vi "Limit Switches.vi"(1 "Mode":enum8{"Start", "Run", "Finish"}(ring)) -> (0 "Limit Switches":T1)   [LabVIEW 2014]
uses:
  <vilib>/Rock Robotics/SystemInterfaces/DIO/FPGA_DIOChannel.ctl
  <vilib>/Rock Robotics/SystemInterfaces/AI/FPGA_AIChannel.ctl
panel:
  out "Voltage":dbl
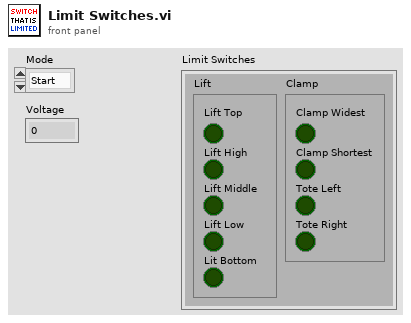
[diagram p1: front panel]
types:
  T1 = cluster{"Lift":cluster{"Lift Top":bool, "Lift High":bool, "Lift Middle":bool, "Lift Low":bool, "Lit Bottom":bool}, "Clamp":cluster{"Clamp Widest":bool, "Clamp Shortest":bool, "Tote Left":bool, "Tote Right":bool}}
  T2 = typedef "FPGA_AIChannel.ctl" = enum8{"AI 0", "AI 1", "AI 2", "AI 3", "AI MXP 0", "AI MXP 1", "AI MXP 2", "AI MXP 3", "Invalid"}
  T3 = typedef "FPGA_DIOChannel.ctl" = enum8{"DIO 0", "DIO 1", "DIO 2", "DIO 3", "DIO 4", "DIO 5", "DIO 6", "DIO 7", "DIO 8", "DIO 9", "DIO MXP 0", "DIO MXP 1", "DIO MXP 2", "DIO MXP 3", "DIO MXP 4", "DIO MXP 5", "DIO MXP 6", "DIO MXP 7", "DIO MXP 8", "DIO MXP 9", "DIO MXP 10", "DIO MXP 11", "DIO MXP 12", "DIO MXP 13", "DIO MXP 14", "DIO MXP 15", "Invalid"}
  T4 = typedef "WPI_AnalogChannelDevRef.ctl" = cluster{"DevStatus":errorcluster, "Controller":T5, "Analog Channel":T2}
  T5 = typedef "FPGA_TypedefAnalogModule.ctl" = enum16{"Controller 1"}
  T6 = typedef "WPI_DigitalInputDevRef.ctl" = cluster{"DevStatus":errorcluster, "DIO Channel":T3, "Controller":T7}
  T7 = typedef "FPGA_TypedefDigitalModule.ctl" = enum16{"Controller 1"}
  T8 = cluster{"Value":bool, "Value":bool, "Value":bool, "Value":bool}
  T9 = cluster{cluster{bool, bool, bool, bool, bool}, cluster{"Value":bool, "Value":bool, "Value":bool, "Value":bool}}
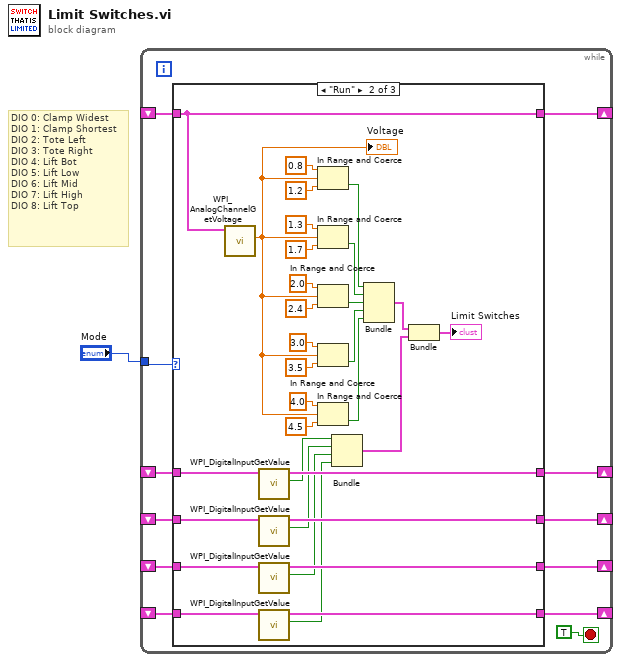
[diagram p0: block diagram]
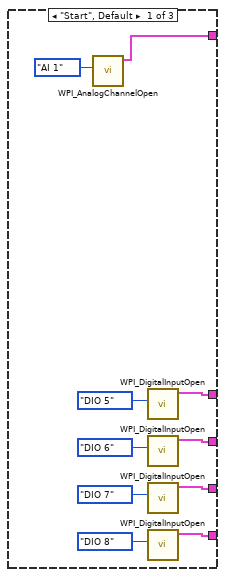
[diagram p2: hidden frame]
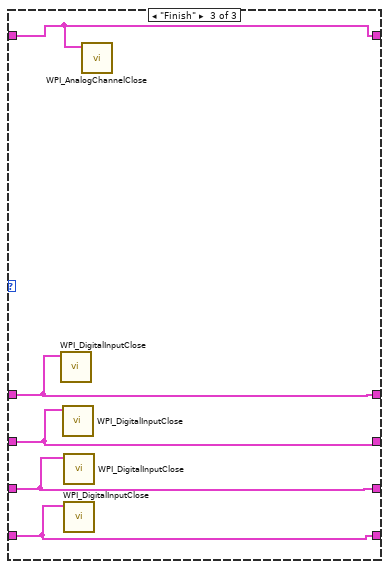
[diagram p3: hidden frame]
diagram:
  # "DIO 0: Clamp Widest\nDIO 1: Clamp Shortest\nDIO 2: Tote Left\nDIO 3: Tote Right\nDIO 4: Lift Bot\nDIO 5: Lift Low\nDIO 6: Lift Mid\nDIO 7: Lift High\nDIO 8: Lift Top"
  n1 = while {
    tunnel: "Mode" -> [w13]
    shift-right: [w12] -> _
    shift-left: _ -> [w11]
    shift-right: [w9] -> _
    shift-left: _ -> [w5]
    shift-right: [w8] -> _
    shift-left: _ -> [w4]
    shift-right: [w7] -> _
    shift-left: _ -> [w3]
    shift-right: [w6] -> _
    shift-left: _ -> [w2]
    stop <- TRUE stop-if-true
    n2 = case shown="\"Run\"" w13 {
      tunnel: [w14 w41 w56] -> w12
      tunnel: w11 -> [_ w41 w56]
      tunnel: [w19 w51 w60] -> w9
      tunnel: [w18 w50 w59] -> w8
      tunnel: [w17 w49 w58] -> w7
      tunnel: [w16 w48 w57] -> w6
      tunnel: w5 -> [_ w55 w60]
      tunnel: w4 -> [_ w54 w59]
      tunnel: w3 -> [_ w53 w58]
      tunnel: w2 -> [_ w52 w57]
      frame "Start", Default {
        n3 = call <vilib>:"WPI_AnalogChannelOpen.vi"("Analog Channel"=FPGA_AIChannel."AI 1") -> ("AIDeviceRef"=w14:T4)  [unwired: 9 in, 1 out]
        n4 = call <vilib>:"WPI_DigitalInputOpen.vi"("DIO Channel"=FPGA_DIOChannel."DIO 5") -> ("DigitalInputDevRef"=w19:T6)  [unwired: 9 in, 1 out]
        n5 = call <vilib>:"WPI_DigitalInputOpen.vi"("DIO Channel"=FPGA_DIOChannel."DIO 6") -> ("DigitalInputDevRef"=w18:T6)  [unwired: 9 in, 1 out]
        n6 = call <vilib>:"WPI_DigitalInputOpen.vi"("DIO Channel"=FPGA_DIOChannel."DIO 7") -> ("DigitalInputDevRef"=w17:T6)  [unwired: 9 in, 1 out]
        n7 = call <vilib>:"WPI_DigitalInputOpen.vi"("DIO Channel"=FPGA_DIOChannel."DIO 8") -> ("DigitalInputDevRef"=w16:T6)  [unwired: 9 in, 1 out]
      }
      frame "Run" {
        n8 = call <vilib>:"WPI_AnalogChannelGetVoltage.vi"("AIDeviceRef"=w41) -> ("Voltage"=w33:dbl)  [unwired: 8 in, 2 out]
        "Voltage" <- w33
        n9 = call <vilib>:"WPI_DigitalInputGetValue.vi"("DigitalInputDevRef"=w55) -> ("Value"=w47:bool, "DigitalInputDevRef"=w51:T6)  [unwired: 8 in, 1 out]
        n10 = call <vilib>:"WPI_DigitalInputGetValue.vi"("DigitalInputDevRef"=w54) -> ("Value"=w46:bool, "DigitalInputDevRef"=w50:T6)  [unwired: 8 in, 1 out]
        n11 = call <vilib>:"WPI_DigitalInputGetValue.vi"("DigitalInputDevRef"=w53) -> ("Value"=w45:bool, "DigitalInputDevRef"=w49:T6)  [unwired: 8 in, 1 out]
        n12 = call <vilib>:"WPI_DigitalInputGetValue.vi"("DigitalInputDevRef"=w52) -> ("Value"=w44:bool, "DigitalInputDevRef"=w48:T6)  [unwired: 8 in, 1 out]
        n13 = In Range and Coerce(upper limit=0.8, x=w33, lower limit=1.2) -> (In Range?=w40:bool)  [unwired: 1 out]
        n14 = In Range and Coerce(upper limit=1.3, x=w33, lower limit=1.7) -> (In Range?=w39:bool)  [unwired: 1 out]
        n15 = In Range and Coerce(upper limit=2.0, x=w33, lower limit=2.4) -> (In Range?=w38:bool)  [unwired: 1 out]
        n16 = In Range and Coerce(upper limit=3.0, x=w33, lower limit=3.5) -> (In Range?=w37:bool)  [unwired: 1 out]
        n17 = In Range and Coerce(upper limit=4.0, x=w33, lower limit=4.5) -> (In Range?=w36:bool)  [unwired: 1 out]
        n18 = Bundle("Value"=w47, "Value"=w46, "Value"=w45, "Value"=w44) -> (w42:T8)  [unwired: 1 in]
        n19 = Bundle(w40, w39, w38, w37, w36) -> (w43:cluster{bool, bool, bool, bool, bool})  [unwired: 1 in]
        n20 = Bundle(w43, w42) -> (→"Limit Switches":T9)  [unwired: 1 in]
      }
      frame "Finish" {
        n21 = call <vilib>:"WPI_DigitalInputClose.vi"("DigitalInputDevRef"=w60) -> ()  [unwired: 10 in, 1 out]
        n22 = call <vilib>:"WPI_DigitalInputClose.vi"("DigitalInputDevRef"=w59) -> ()  [unwired: 10 in, 1 out]
        n23 = call <vilib>:"WPI_DigitalInputClose.vi"("DigitalInputDevRef"=w58) -> ()  [unwired: 10 in, 1 out]
        n24 = call <vilib>:"WPI_DigitalInputClose.vi"("DigitalInputDevRef"=w57) -> ()  [unwired: 10 in, 1 out]
        n25 = call <vilib>:"WPI_AnalogChannelClose.vi"("AIDeviceRef"=w56) -> ()  [unwired: 10 in, 1 out]
      }
    }
  }
